vi "Multiply Two Numbers.vi"(10 "Numeric 2":dbl, 11 "Numeric":dbl) -> (3 "Numeric 3":dbl)   [LabVIEW 2010, in "TopNamespace.lvlib" / "SubNamespace.lvlib"]
uses:
  SubNamespace.lvlib
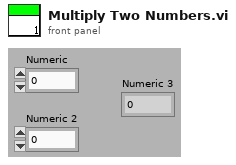
[diagram p1: front panel]
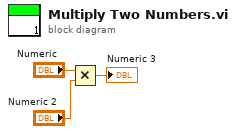
[diagram p0: block diagram]
diagram:
  n1 = Multiply(x="Numeric", y="Numeric 2") -> (x*y=→"Numeric 3":dbl)
